vi "niDTS WLAN DSSS Tx Test UTIL WLAN to DSSS ModAcc Settings.vi"(9 "ModAcc DSSS Paramaters":T1={"DC Offset Compensation"=TRUE, "Equalization"=TRUE, "Phase Tracking"=TRUE, "Chip Start Location"=0, "Max Chips Used"=16, "Pulse Shaping FilterType"=enum."GAUSSIAN", "Pulse Shaping Filter Coefficient"=0.35}, 10 "ModAcc Measurement Paramaters":T4={"ModAcc Enable"=FALSE, "Header Detection"=enum."FIRST", "Averages"=3, "Amplitude Tracking"=FALSE, "Channel Tracking"=FALSE, "Time Tracking"=TRUE, "Phase Tracking"=enum."NONE", "Clock Offset Est"=FALSE, "Impairments Est"=FALSE, "CFO Estimation"=enum."PAMBLE"}) -> (2 "DSSS ModAcc Measurement Paramaters":T3={"ModAcc Enable"=FALSE, "Header Detection"=enum."FIRST", "Averages"=0, "CFO Estimation"=enum."PAMBLE", "DC Offset Compensation"=FALSE, "Chip Start Location"=0, "Max Chips Used"=16, "Pulse Shaping FilterType"=enum."NONE", "Pulse Shaping Filter Coefficient"=0.35, "Equalization"=FALSE, "Phase Tracking"=TRUE})   [LabVIEW 2014, in "niDTS WLAN.lvlib"]
uses:
  niDTS WLAN.lvlib
  Includes/niDTS WLAN INC ModAcc Measurement Parameters.ctl
  Includes/niDTS WLAN DSSS Tx Test INC ModAcc Measurement Parameters.ctl
  Includes/niDTS WLAN INC Pulse Shaping Filter Type.ctl
  Includes/niDTS WLAN INC DSSS ModAcc Measurement Parameters.ctl
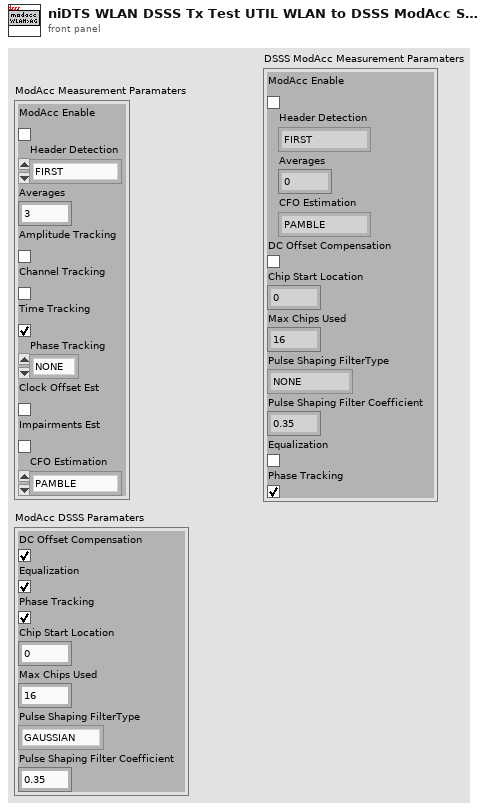
[diagram p1: front panel]
types:
  T1 = typedef "niDTS WLAN.lvlib/niDTS WLAN INC DSSS ModAcc Measurement Parameters.ctl" = cluster{"DC Offset Compensation":bool, "Equalization":bool, "Phase Tracking":bool, "Chip Start Location":i16, "Max Chips Used":i16, "Pulse Shaping FilterType":T2, "Pulse Shaping Filter Coefficient":dbl}
  T2 = typedef "niDTS WLAN.lvlib/niDTS WLAN INC Pulse Shaping Filter Type.ctl" = enum16{"NONE", "RCOSINE", "RRCOSINE", "GAUSSIAN"}
  T3 = typedef "niDTS WLAN.lvlib/niDTS WLAN DSSS Tx Test INC ModAcc Measurement Parameters.ctl" = cluster{"ModAcc Enable":bool, "Header Detection":enum16{"MANUAL", "FIRST", "ALL"}, "Averages":i32, "CFO Estimation":enum16{"PAMBLE", "PDATA"}, "DC Offset Compensation":bool, "Chip Start Location":i16, "Max Chips Used":i16, "Pulse Shaping FilterType":T2, "Pulse Shaping Filter Coefficient":dbl, "Equalization":bool, "Phase Tracking":bool}
  T4 = typedef "niDTS WLAN.lvlib/niDTS WLAN INC ModAcc Measurement Parameters.ctl" = cluster{"ModAcc Enable":bool, "Header Detection":enum16{"MANUAL", "FIRST", "ALL"}, "Averages":i32, "Amplitude Tracking":bool, "Channel Tracking":bool, "Time Tracking":bool, "Phase Tracking":enum16{"NONE", "STANDARD", "CSF", "INSTANT"}, "Clock Offset Est":bool, "Impairments Est":bool, "CFO Estimation":enum16{"PAMBLE", "PDATA"}}
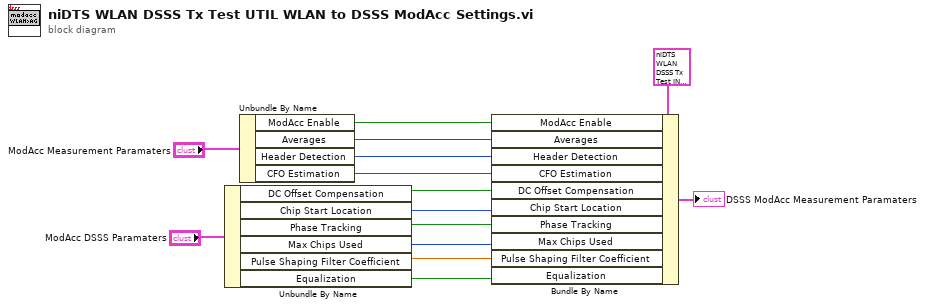
[diagram p0: block diagram]
diagram:
  n1 = Unbundle By Name("ModAcc DSSS Paramaters") -> ("DC Offset Compensation"=w6:bool, "Chip Start Location"=w5:i16, "Phase Tracking"=w4:bool, "Max Chips Used"=w3:i16, "Pulse Shaping Filter Coefficient"=w2:dbl, "Equalization"=w1:bool)
  n2 = Unbundle By Name("ModAcc Measurement Paramaters") -> ("ModAcc Enable"=w11:bool, "Averages"=w14:i32, "Header Detection"=w10:enum16{"MANUAL", "FIRST", "ALL"}, "CFO Estimation"=w13:enum16{"PAMBLE", "PDATA"})
  n3 = Bundle By Name(cluster=T3 {"ModAcc Enable"=FALSE, "Header Detection"=enum."FIRST", "Averages"=0, "CFO Estimation"=enum."PAMBLE", "DC Offset Compensation"=FALSE, "Chip Start Location"=0, "Max Chips Used"=16, "Pulse Shaping FilterType"=enum."NONE", "Pulse Shaping Filter Coefficient"=0.35, "Equalization"=FALSE, "Phase Tracking"=TRUE} ("DSSS ModAcc Measurement Paramaters"), "ModAcc Enable"=w11, "Averages"=w14, "Header Detection"=w10, "CFO Estimation"=w13, "DC Offset Compensation"=w6, "Chip Start Location"=w5, "Phase Tracking"=w4, "Max Chips Used"=w3, "Pulse Shaping Filter Coefficient"=w2, "Equalization"=w1) -> (→"DSSS ModAcc Measurement Paramaters":T3)
